vi "Init.vi"(8 "error in":errorcluster, 11 "MyTestHeader in":refnum<class "MyTestHeader.lvclass">) -> (0 "error out":errorcluster, 3 "MyTestHeader out":refnum<class "MyTestHeader.lvclass">)   [LabVIEW 2023, in "MyTestHeader.lvclass"]
uses:
  MyTestHeader.lvclass
  source/Views/ColumnHeader View/ColumnHeader View.lvclass
  source/Cells/ColumnHeader/Column Header.lvclass
  source/Font/Font.lvclass
  source/System.Drawing.Color.ctl
  source/SourceGrid.lvlib
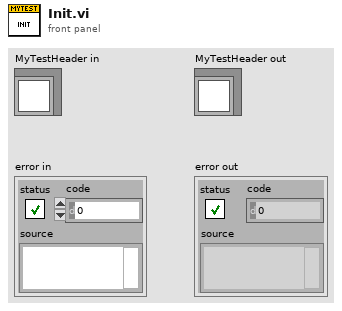
[diagram p1: front panel]
types:
  T1 = typedef "SourceGrid.lvlib/System.Drawing.Color.ctl" = enum16{"AliceBlue", "AntiqueWhite", "Aqua", "Aquamarine", "Azure", "Beige", "Bisque", "Black", "BlanchedAlmond", "Blue", "BlueViolet", "Brown", "BurlyWood", "CadetBlue", "Chartreuse", "Chocolate", "Coral", "CornflowerBlue", "Cornsilk", "Crimson", "Cyan", "DarkBlue", "DarkCyan", "DarkGoldenrod", "DarkGray", "DarkGreen", "DarkKhaki", "DarkMagenta", "DarkOliveGreen", "DarkOrange", "DarkOrchid", "DarkRed", "DarkSalmon", "DarkSeaGreen", "DarkSlateBlue", "DarkSlateGray", "DarkTurquoise", "DarkViolet", "DeepPink", "DeepSkyBlue", "DimGray", "DodgerBlue", "Firebrick", "FloralWhite", "ForestGreen", "Fuchsia", "Gainsboro", "GhostWhite", "Gold", "Goldenrod", "Gray", "Green", "GreenYellow", "Honeydew", "HotPink", "IndianRed", "Indigo", "Ivory", "Khaki", "Lavender", "LavenderBlush", "LawnGreen", "LemonChiffon", "LightBlue", "LightCoral", "LightCyan", "LightGoldenrodYellow", "LightGray", "LightGreen", "LightPink", "LightSalmon", "LightSeaGreen", "LightSkyBlue", "LightSlateGray", "LightSteelBlue", "LightYellow", "Lime", "LimeGreen", "Linen", "Magenta", "Maroon", "MediumAquamarine", "MediumBlue", "MediumOrchid", "MediumPurple", "MediumSeaGreen", "MediumSlateBlue", "MediumSpringGreen", "MediumTurquoise", "MediumVioletRed", "MidnightBlue", "MintCream", "MistyRose", "Moccasin", "NavajoWhite", "Navy", "OldLace", "Olive", "OliveDrab", "Orange", "OrangeRed", "Orchid", "PaleGoldenrod", "PaleGreen", "PaleTurquoise", "PaleVioletRed", "PapayaWhip", "PeachPuff", "Peru", "Pink", "Plum", "PowderBlue", "Purple", "Red", "RosyBrown", "RoyalBlue", "SaddleBrown", "Salmon", "SandyBrown", "SeaGreen", "SeaShell", "Sienna", "Silver", "SkyBlue", "SlateBlue", "SlateGray", "Snow", "SpringGreen", "SteelBlue", "Tan", "Teal", "Thistle", "Tomato", "Transparent", "Turquoise", "Violet", "Wheat", "White", "WhiteSmoke", "Yellow"}
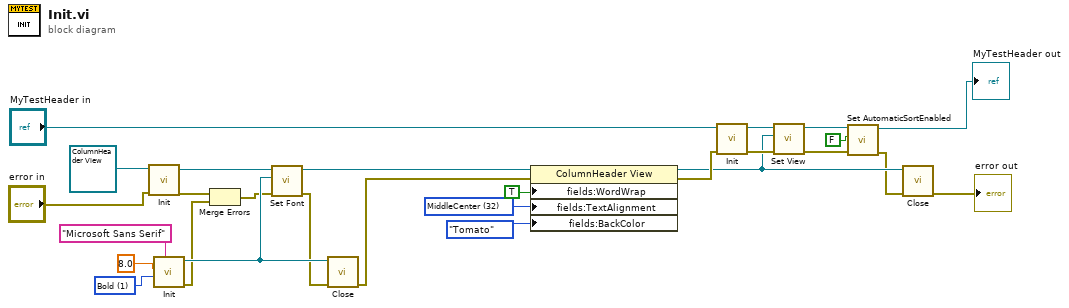
[diagram p0: block diagram]
diagram:
  w17 = 32 items=["TopLeft"=1, "TopCenter"=2, "TopRight"=4, "MiddleLeft"=16, "MiddleCenter"=32, "MiddleRight"=64, "BottomLeft"=256, "BottomCenter"=512, "BottomRight"=1024] ("TextAlignment")
  w21 = 1 items=["Regular"=0, "Bold"=1, "Italic"=2, "Underline"=4, "Strikeout"=8] ("style")
  n1 = call-dynamic "Init.vi"("error in"="error in", "ColumnHeader View in"=refnum<class "ColumnHeader View.lvclass"> refnum ("ColumnHeader View")) -> ("error out"=w19:errorcluster, "ColumnHeader View out"=w24:refnum<class "ColumnHeader View.lvclass">)  [unwired: 8 in]
  n2 = call "Init.vi"("family"="Microsoft Sans Serif", "style"=w21, "emSize"=sgl 8.0) -> ("error out"=w5:errorcluster, "Font out"=w7:refnum<class "Font.lvclass">)  [unwired: 7 in]
  n3 = Merge Errors(w19, w5) -> (w6:errorcluster)
  n4 = call-dynamic "Set Font.vi"("error in"=w6, "Font.lvclass"=w7, "View in"=w24) -> ("error out"=w4:errorcluster, "View out"=w20:refnum<class "ColumnHeader View.lvclass">)  [unwired: 7 in]
  n5 = call-dynamic "Close.vi"("error in"=w4, "Font in"=w7) -> ("error out"=w8:errorcluster)  [unwired: 8 in, 1 out]
  n6 = property class="ColumnHeader View"(reference=w20, error in=w8, "fields:WordWrap"=TRUE ("WordWrap"), "fields:TextAlignment"=w17, "fields:BackColor"=System.Drawing.Color."Tomato" ("BackColor")) -> (reference out=w3:refnum<class "ColumnHeader View.lvclass">, error out=w14:errorcluster)
  n7 = call-parent "Init.vi"("error in"=w14, "Column Header in"="MyTestHeader in") -> ("error out"=w27:errorcluster, "Column Header out"=w16:refnum<class "MyTestHeader.lvclass">)  [unwired: 8 in]
  n8 = call-dynamic "Set View.vi"("error in"=w27, "CellView"=w3, "Cell in"=w16) -> ("error out"=w11:errorcluster, "Cell out"=w13:refnum<class "MyTestHeader.lvclass">)  [unwired: 7 in]
  n9 = call "Set AutomaticSortEnabled.vi"("error in"=w11, "AutomaticSortEnabled"=FALSE, "ColumnHeader in"=w13) -> ("error out"=w2:errorcluster, "ColumnHeader out"=→"MyTestHeader out":refnum<class "MyTestHeader.lvclass">)  [unwired: 7 in]
  n10 = call-dynamic "Close.vi"("error in"=w2, "Cell View in"=w3) -> ("error out"=→"error out":errorcluster)  [unwired: 8 in, 1 out]
